vi "roi index.vi"(10 "Value":dbl format="%#_13g", 11 "Data":dbl[](array[numeric])) -> (3 "Minimum Element":i32)   [LabVIEW 2023]
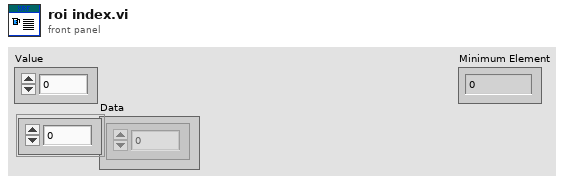
[diagram p1: front panel]
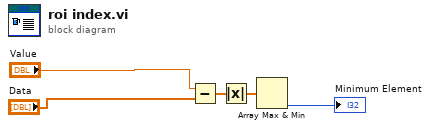
[diagram p0: block diagram]
diagram:
  n1 = Subtract(x="Value", y="Data") -> (x-y=w3:dbl[])
  n2 = Absolute Value(x=w3) -> (abs(x)=w2:dbl[])
  n3 = Array Max & Min(array=w2) -> (min index (indices)=→"Minimum Element":i32)  [unwired: 3 out]
